vi "CD Init_Prepare Inline Data_Fill In BC part of Frame Descriptor.vi"(11 "message":T8 {"Timestamp Channel Data Reference" format="%.0x"; "Status Channel Data Refs" format="%.0x"; "param item refs" format="%.0x"; "param Block Data Refs"."Data Reference" format="%.0x"}) -> (3 "BC Frame Descriptor":T1 {"Status Channel Refs" format="%.0x"; "param block data refs"."Data Reference" format="%.0x"; "Timestamp Channel Data Reference" format="%.0x"})   [LabVIEW 2020, in "Ballard MIL-1553 Engine.lvlib"]
uses:
  Ballard MIL-1553 Engine.lvlib
  Shared/Controls and Global/RT Message.ctl
  Shared/Controls and Global/RT messageType.ctl
  Shared/Controls and Global/RT CWD1.ctl
  Shared/Controls and Global/RT CWD2.ctl
  <vilib>/NI VeriStand/Custom Device API/Data Reference.ctl
  <vilib>/NI VeriStand/Custom Device API/Custom Device Item Ref.ctl
  <vilib>/NI VeriStand/Custom Device API/Block Data Reference.ctl
  System Explorer/SubVIs/Parse Parameters File/param_map_sysdef_type.ctl
  Azdo/emea-ni-vscd_Configurator/source/ConfiguratorConsumer/Helpers/Configuration/_typedefs/param_type.ctl
  Azdo/emea-ni-vscd_Configurator/source/ConfiguratorConsumer/Helpers/Configuration/_typedefs/param_signalType_type.ctl
  Azdo/emea-ni-vscd_Configurator/source/ConfiguratorConsumer/Helpers/Configuration/_typedefs/param_encoding_type.ctl
  Controls/RT Inline Frame Descriptor_BC.ctl
  Shared/EncodeDecode/_typedefs/parameter_config_type.ctl
  Shared/EncodeDecode/_typedefs/parameter_config_type_type.ctl
  Shared/EncodeDecode/_typedefs/parameter_config_encoding_type.ctl
  <vilib>/NI VeriStand/Custom Device API/Custom Device API.lvlib
  Shared/Ballard 1553 Shared.lvlib
  Azdo/emea-ni-vscd_Configurator/source/ConfiguratorConsumer/Helpers/Configuration/Configuration_Helper.lvlib
  System Explorer/Ballard 1553 System Explorer.lvlib
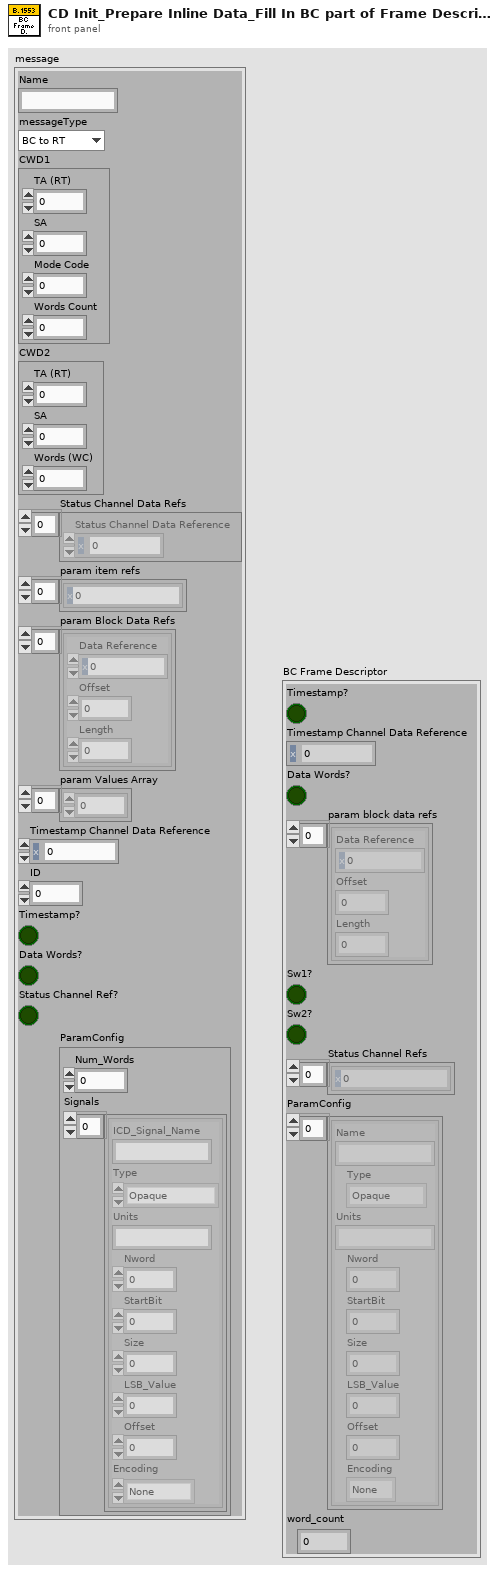
[diagram p1: front panel]
types:
  T1 = typedef "Ballard MIL-1553 Engine.lvlib/RT Inline Frame Descriptor_BC.ctl" = cluster{"Timestamp?":bool, "Timestamp Channel Data Reference":T2, "Data Words?":bool, "param block data refs":T3[], "Sw1?":bool, "Sw2?":bool, "Status Channel Refs":T4[], "ParamConfig":T5[], "word_count":u8}
  T2 = typedef "Custom Device API.lvlib/Data Reference.ctl" = i32
  T3 = typedef "Custom Device API.lvlib/Block Data Reference.ctl" = cluster{"Data Reference":T2, "Offset":u64, "Length":u64}
  T4 = typedef "Custom Device API.lvlib/Custom Device Item Ref.ctl" = u64
  T5 = typedef "parameter_config_type.ctl" = cluster{"Name":string, "Type":T6, "Units":string, "Nword":i32, "StartBit":i32, "Size":i32, "LSB_Value":dbl, "Offset":i32, "Encoding":T7}
  T6 = typedef "parameter_config_type_type.ctl" = enum16{"Opaque", "Enum", "Float", "Integer", "Bcd", "Bool"}
  T7 = typedef "parameter_config_encoding_type.ctl" = enum16{"None", "2-complement", "Unsigned"}
  T8 = typedef "Ballard 1553 Shared.lvlib/RT Message.ctl" = cluster{"Name":string, "messageType":T9, "CWD1":T10, "CWD2":T11, "Status Channel Data Refs":T2[], "param item refs":T4[], "param Block Data Refs":T3[], "param Values Array":u16[], "Timestamp Channel Data Reference":T2, "ID":i32, "Timestamp?":bool, "Data Words?":bool, "Status Channel Ref?":bool, "ParamConfig":T12}
  T9 = typedef "Ballard 1553 Shared.lvlib/RT messageType.ctl" = enum16{"BC to RT", "RT to BC", "RT to RT", "MC (Rx)", "MC (Tx)"}
  T10 = typedef "Ballard 1553 Shared.lvlib/RT CWD1.ctl" = cluster{"TA (RT)":i8, "SA":i8, "Mode Code":i8, "Words Count":i8}
  T11 = typedef "Ballard 1553 Shared.lvlib/RT CWD2.ctl" = cluster{"TA (RT)":i8, "SA":i8, "Words (WC)":i8}
  T12 = typedef "Ballard 1553 System Explorer.lvlib/param_map_sysdef_type.ctl" = cluster{"Num_Words":u8, "Signals":T13[]}
  T13 = typedef "Configuration_Helper.lvlib/param_type.ctl" = cluster{"ICD_Signal_Name":string, "Type":T14, "Units":string, "Nword":i32, "StartBit":i32, "Size":i32, "LSB_Value":dbl, "Offset":i32, "Encoding":T15}
  T14 = typedef "Configuration_Helper.lvlib/param_signalType_type.ctl" = enum16{"Opaque", "Enum", "Float", "Integer", "Bcd", "Bool"}
  T15 = typedef "Configuration_Helper.lvlib/param_encoding_type.ctl" = enum16{"None", "2-complement", "Unsigned"}
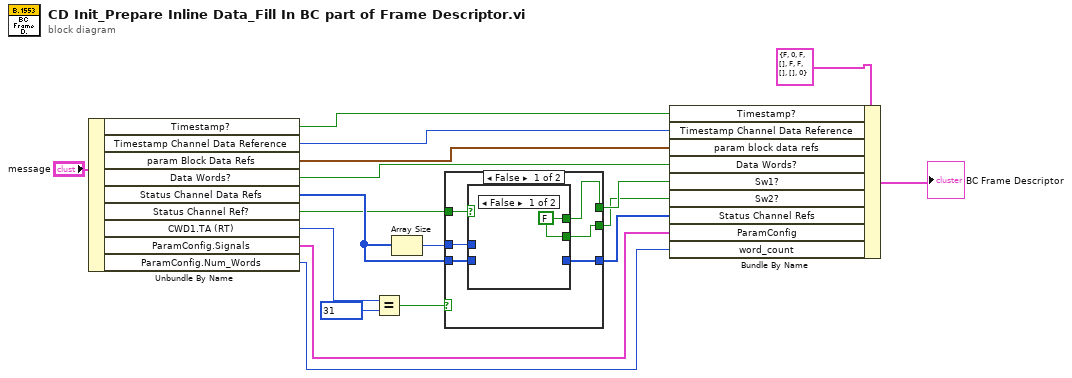
[diagram p0: block diagram]
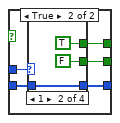
[diagram p2: hidden frame]
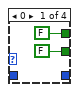
[diagram p3: hidden frame]
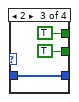
[diagram p4: hidden frame]
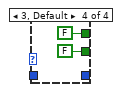
[diagram p5: hidden frame]
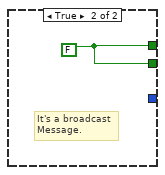
[diagram p6: hidden frame]
diagram:
  n1 = Unbundle By Name("message") -> ("Timestamp?"=w9:bool, "Timestamp Channel Data Reference"=w17:T2, "param Block Data Refs"=w16:T3[], "Data Words?"=w7:bool, "Status Channel Data Refs"=w8:T2[], "Status Channel Ref?"=w5:bool, "CWD1.TA (RT)"=w6:i8, "ParamConfig.Signals"=w4:T13[], "ParamConfig.Num_Words"=w3:u8)
  n2 = Equal?(x=w6, y=i8 31) -> (x = y?=w10:bool)
  n3 = Array Size(array=w8) -> (size(s)=w15:i32)
  n4 = case shown="False" w10 {
    tunnel: w15 -> [w24 _]
    tunnel: [w23 w41] -> w14
    tunnel: [w22 w41] -> w13
    tunnel: w8 -> [w21 _]
    tunnel: [w20 _] -> w12
    tunnel: w5 -> [w19 _]
    frame False {
      n5 = case shown="False" w19 {
        tunnel: w24 -> [_ w30]
        tunnel: [w25 w29] -> w23
        tunnel: [w25 w28] -> w22
        tunnel: w21 -> [_ w27]
        tunnel: [_ w26] -> w20
        frame False {
          w25 = FALSE
        }
        frame True {
          n6 = case shown="1" w30 {
            tunnel: [FALSE TRUE TRUE FALSE] -> w29
            tunnel: [FALSE FALSE TRUE FALSE] -> w28
            tunnel: w27 -> [_ w33 w36 _]
            tunnel: [_ w33 w36 _] -> w26
            frame 0 {
            }
            frame 1 {
            }
            frame 2 {
            }
            frame 3, Default {
            }
          }
        }
      }
    }
    frame True {
      w41 = FALSE
      # "It's a broadcast\nMessage."
    }
  }
  n7 = Bundle By Name(cluster=T1 {"Timestamp?"=FALSE, "Timestamp Channel Data Reference"=0, "Data Words?"=FALSE, "param block data refs"=[], "Sw1?"=FALSE, "Sw2?"=FALSE, "Status Channel Refs"=[], "ParamConfig"=[], "word_count"=0} ("BC"), "Timestamp?"=w9, "Timestamp Channel Data Reference"=w17, "param block data refs"=w16, "Data Words?"=w7, "Sw1?"=w14, "Sw2?"=w13, "Status Channel Refs"=w12, "ParamConfig"=w4, "word_count"=w3) -> (→"BC Frame Descriptor":T1)
